vi "HAL camera error handler.vi"(8 "error in (no error)":errorcluster) -> (0 "error out":errorcluster)   [LabVIEW 2016]
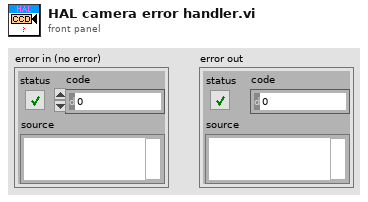
[diagram p1: front panel]
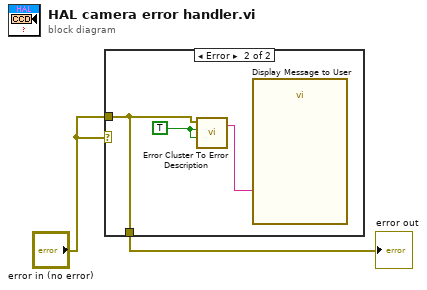
[diagram p0: block diagram]
diagram:
  n1 = case shown="Error" "error in (no error)" {
    tunnel: "error in (no error)" -> [w3 w4]
    tunnel: [w3 w4] -> w2
    frame No Error {
    }
    frame Error {
      w6 = TRUE ("show name (F)")
      n2 = call <userlib>:"Error Cluster To Error Description.vi"("show DLL error code (F)"=w6, "show name (F)"=w6, "error cluster"=w4) -> ("description"=w5:string)  [unwired: 1 in, 1 out]
      n3 = call "Display Message to User"("Message"=w5) -> ()  [unwired: 9 in, 2 out]
    }
  }
  "error out" <- w2
